vi "CommitSettings.vi"(1 "SmartScope in":refnum<k24>) -> (0 "SmartScope out":refnum<k24>)   [LabVIEW 2019]
uses:
  C:/Program Files (x86)/LabNation/SmartScope/DeviceInterface.dll
  Program Files (x86)/LabNation/SmartScope/DeviceInterface.dll
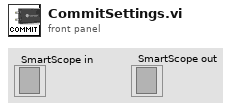
[diagram p1: front panel]
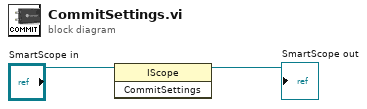
[diagram p0: block diagram]
diagram:
  n1 = invoke class="IScope" method="CommitSettings"(reference="SmartScope in") -> (reference out=→"SmartScope out":refnum<k24>)  [unwired: 2 in, 2 out]
